vi "Temperature.vi"(0 "physical channels":tag="PXI1Slot2/ai2", 1 "current excitation value":dbl=0.0009 format="%0.5f", 2 "r0":dbl=100.0 format="%0.2f", 5 "current excitation source":i32(ring)=10200 items=["Internal"=10200, "External"=10167, "None"=10230], 7 "resistance configuration":i32(ring)=2 items=["2-Wire"=2, "3-Wire"=3, "4-Wire"=4], 9 "rtd type":i32(ring)=10071 items=["Pt3750"=12481, "Pt3851"=10071, "Pt3911"=12482, "Pt3916"=10069, "Pt3920"=10053, "Pt3928"=12483, "Custom"=10137], 11 "units":i32(ring)=10143 items=["Deg C"=10143, "Deg F"=10144, "Kelvins"=10325, "Deg R"=10145, "From Custom Scale"=10065], 12 "minimum value":dbl format="%0.2f", 13 "maximum value":dbl=100.0 format="%0.2f") -> (4 "data":dbl[](array[numeric]) format="%0.2f", 8 "spreadsheet string":string, 15 "error out":errorcluster)   [LabVIEW 2019]
uses:
  <vilib>/DAQmx/read.llb/DAQmx Read (Analog 1D DBL NChan 1Samp).vi
  <vilib>/DAQmx/create/channels.llb/DAQmx Create Channel (AI-Temperature-RTD).vi
  <vilib>/DAQmx/miscellaneous.llb/DAQmx Fill In Error Info.vi
panel:
  # "Para el NI PXIe-4357"
  # "chanel 2 (ai2) for rtd"
  # "Pt3851 for rtd"
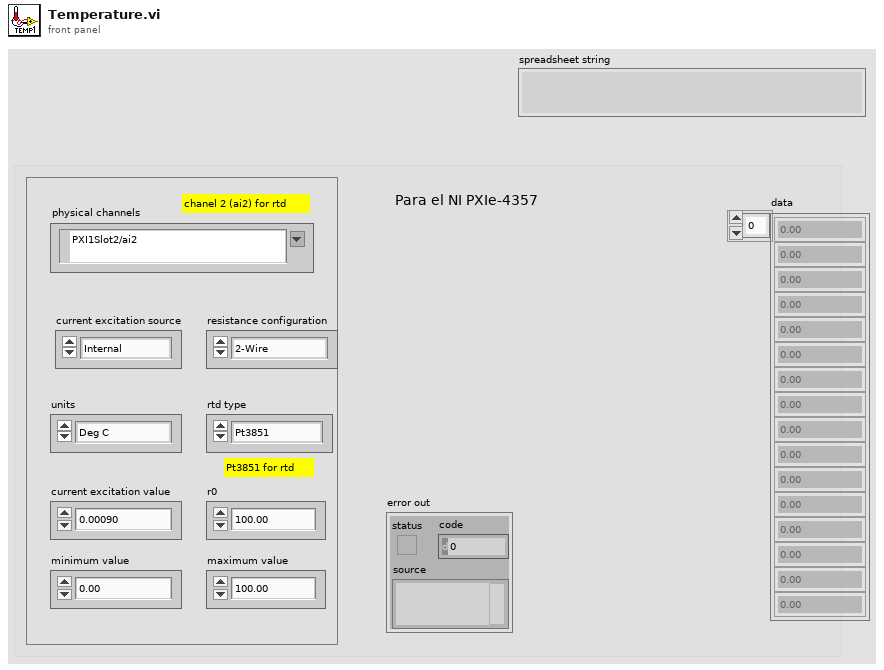
[diagram p1: front panel]
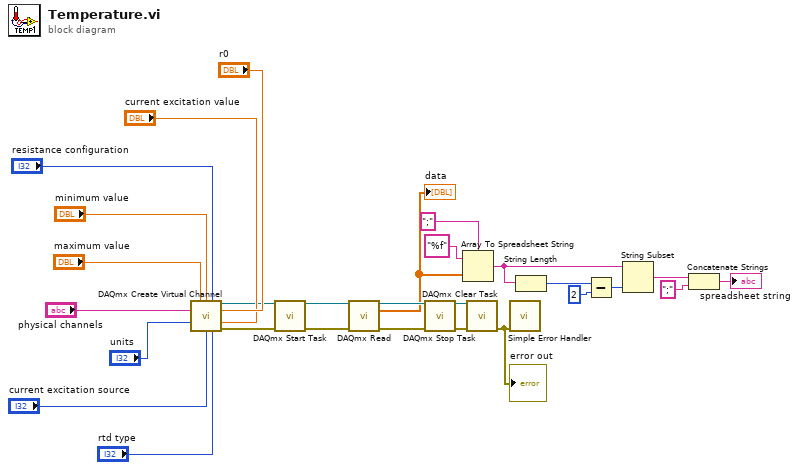
[diagram p0: block diagram]
diagram:
  n1 = call-poly <vilib>:"DAQmx Create Virtual Channel.vi"("maximum value"="maximum value", "minimum value"="minimum value", "resistance configuration"="resistance configuration", "physical channels"="physical channels", "r0"="r0", "units"="units", "current excitation value"="current excitation value", "current excitation source"="current excitation source", "rtd type"="rtd type") -> ("task out"=w9:refnum<k21>, "error out"=w10:errorcluster)  [unwired: 5 in]
  n2 = call <vilib>:"DAQmx Start Task.vi"("task/channels in"=w9, "error in"=w10) -> ("task out"=w15:refnum<k21>, "error out"=w16:errorcluster)  [unwired: 12 in]
  n3 = call-poly <vilib>:"DAQmx Read.vi"("task/channels in"=w15, "error in"=w16) -> ("task out"=w17:refnum<k21>, "data"=w8:dbl[], "error out"=w18:errorcluster)  [unwired: 11 in]
  "data" <- w8
  n4 = call <vilib>:"DAQmx Stop Task.vi"("task/channels in"=w17, "error in"=w18) -> ("task out"=w14:refnum<k21>, "error out"=w13:errorcluster)  [unwired: 12 in]
  n5 = Array To Spreadsheet String(delimiter (Tab)=";", array=w8, 3:"%f" ("format string")) -> (spreadsheet string=w7:string)
  n6 = call <vilib>:"DAQmx Clear Task.vi"("task in"=w14, "error in"=w13) -> ("error out"=w28:errorcluster)  [unwired: 13 in]
  "error out" <- w28
  n7 = call <vilib>:"Simple Error Handler.vi"("error in (no error)"=w28) -> ()  [unwired: 4 in, 5 out]
  n8 = String Length(string=w7) -> (length=w6:i32)
  n9 = Subtract(x=w6, y=2) -> (x-y=w4:i32)
  n10 = String Subset(string=w7, length (rest)=w4) -> (substring=w3:string)  [unwired: 1 in]
  n11 = Concatenate Strings(w3, ";" ("string")) -> (→"spreadsheet string":string)
